vi "OrbitData.vi"(1 "e":dbl, 2 "a":dbl) -> (0 "Orbit XY":cluster{dbl[], dbl[]})   [LabVIEW 2020]
doc: "Returns object orbit as a cluster of X and Y array."
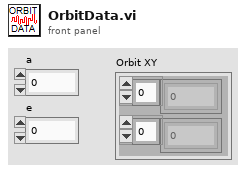
[diagram p1: front panel]
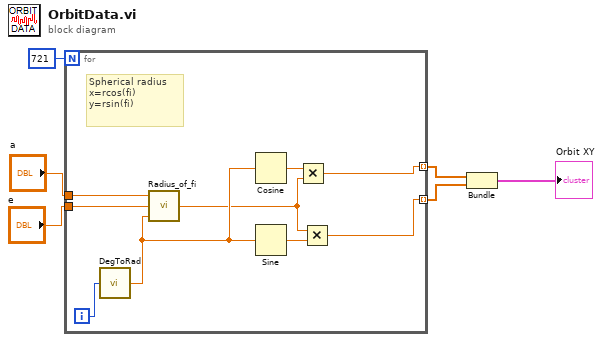
[diagram p0: block diagram]
diagram:
  n1 = for {
    N: 721 -> [_]
    tunnel: [w9] -> w6 mode=indexing
    tunnel: [w8] -> w5 mode=indexing
    tunnel: "a" -> [w11]
    tunnel: "e" -> [w10]
    i -> [w7]
    # "Spherical radius\nx=rcos(fi)\ny=rsin(fi)"
    n2 = call "DegToRad.vi"("fi in degrees"=w7) -> ("fi in radians"=w15:dbl)
    n3 = call "Radius_of_fi.vi"("fi"=w15, "e"=w10, "a"=w11) -> ("r"=w14:dbl)
    n4 = Cosine(x=w15) -> (cos(x)=w13:dbl)
    n5 = Sine(x=w15) -> (sin(x)=w12:dbl)
    n6 = Multiply(x=w13, y=w14) -> (x*y=w8:dbl)
    n7 = Multiply(x=w14, y=w12) -> (x*y=w9:dbl)
  }
  n8 = Bundle(w5, w6) -> (→"Orbit XY":cluster{dbl[], dbl[]})  [unwired: 1 in]
